vi "AD Detect Lv3 Motor Disconnect SPARKMAX.vi"(2 "Items Out":string[](array[string]), 3 "String":string) -> (0 "Array 2":bool[](array[boolean]), 1 "Array":string[](array[string]))   [LabVIEW 2019]
uses:
  <vilib>/Rock Robotics/WPI/ThirdParty/REV Robotics/SPARK MAX/Typedef/Spark MAX CAN API Mask.ctl
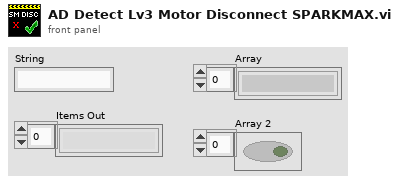
[diagram p1: front panel]
types:
  T1 = typedef "Spark MAX CAN API Mask.ctl" = u32
  T2 = typedef "WPI_MotorControlDeviceRef.ctl" = cluster{"DeviceStatus":errorcluster, "Type":T3, "PWM":cluster{"PWM Channel":T4, "DeadBand":T5}, "CAN":cluster{"Device Number":u8, "SetOutput VI Ref":variant, "GetOutput VI Ref":variant, "Enable VI Ref":variant, "Disable VI Ref":variant, "Data":variant}, "Invert":bool, "DIO PWM":cluster{"PWM \"Enable\" Channel":T4, "DIOChannel":T6, "PWM Rate":dbl}}
  T3 = typedef "WPI_MotorControlType.ctl" = enum16{"PWM", "CAN", "DIO PWM"}
  T4 = typedef "FPGA_DIOPWMChannel.ctl" = enum8{"PWM 0", "PWM 1", "PWM 2", "PWM 3", "PWM 4", "PWM 5", "PWM 6", "PWM 7", "PWM 8", "PWM 9", "PWM MXP 0", "PWM MXP 1", "PWM MXP 2", "PWM MXP 3", "PWM MXP 4", "PWM MXP 5", "PWM MXP 6", "PWM MXP 7", "PWM MXP 8", "PWM MXP 9", "Invalid"}
  T5 = typedef "WPI_PWMDeadband.ctl" = cluster{"Name":string, "maxPositivePwm":i32, "minPositivePwm":i32, "centerPwm":i32, "maxNegativePwm":i32, "minNegativePwm":i32, "angularRange":u16}
  T6 = typedef "FPGA_DIOChannel.ctl" = enum8{"DIO 0", "DIO 1", "DIO 2", "DIO 3", "DIO 4", "DIO 5", "DIO 6", "DIO 7", "DIO 8", "DIO 9", "DIO MXP 0", "DIO MXP 1", "DIO MXP 2", "DIO MXP 3", "DIO MXP 4", "DIO MXP 5", "DIO MXP 6", "DIO MXP 7", "DIO MXP 8", "DIO MXP 9", "DIO MXP 10", "DIO MXP 11", "DIO MXP 12", "DIO MXP 13", "DIO MXP 14", "DIO MXP 15", "SPI Port CS1", "SPI Port CS2", "SPI Port CS3", "SPI Port MISO", "SPI Port MOSI", "Invalid"}
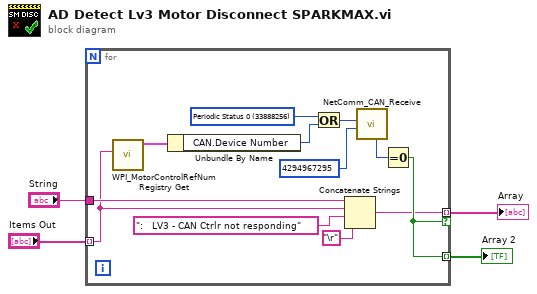
[diagram p0: block diagram]
diagram:
  n1 = for {
    tunnel: "Items Out" -> [w5] mode=indexing
    tunnel: [w7] -> w2 mode=indexing if=w8
    tunnel: [w8] -> w1 mode=indexing
    tunnel: "String" -> [w6]
    w12 = T1 33888256 items=["Broadcast Disable"=0, "Broadcast System Halt"=64, "Broadcast System Reset"=128, "Broadcast Device Assign"=192, "Broadcast Heartbeat"=320, "Broadcast Firmware Version"=512, "Broadcast Enumerate"=576, "Broadcast System Resume"=640, "Setpoint Set"=33882176, "Duty Cycle Set"=33882240, "Speed Set"=33883264, "Position Set"=33885312, "Voltage Set"=33886336, "Periodic Status 0"=33888256, "Periodic Status 1"=33888320, "Periodic Status 2"=33888384, "User Status 0"=33888448, "User Status 1"=33888512, "User Status 2"=33888576, "DRV Status"=33888896, "Clear Faults"=33889152, "Set Config Parameter"=33889280, "Get Config Parameter"=33889344, "Config Burn Flash"=33889408, "Set Follower Mode"=33889472, "Nack"=33890304, "Ack"=33890368, "Heartbeat"=33891456, "Sync"=33891520, "IDQuery"=33891584, "IDAssign"=33891648, "Firmware Version"=33891840] ("Parameter ID")
    n2 = call <vilib>:"WPI_MotorControlRefNum Registry Get.vi"("refnum name"=w5) -> ("MotorControlDevRef"=w14:T2)  [unwired: 9 in, 1 out]
    n3 = Unbundle By Name(w14) -> ("CAN.Device Number"=w15:u8)
    n4 = Or(x=w12, y=w15) -> (x .or. y?=w16:T1)
    n5 = Concatenate Strings(w6, w5, ":   LV3 - CAN Ctrlr not responding", "\r") -> (w7:string)
    n6 = call <vilib>:"NetComm_CAN_Receive.vi"("Message ID Mask"=u32 4294967295, "Message ID"=w16) -> ("timeStamp"=w9:u32)  [unwired: 1 in, 8 out]
    n7 = Equal To 0?(x=w9) -> (x = 0?=w8:bool)
  }
  "Array" <- w2
  "Array 2" <- w1
